vi "Upload Firmware.vi"(5 "Progress Bar":refnum<vi>, 7 "COM Port":refnum<visa-resource-name>="COM5", 8 "Error In":errorcluster, 9 "Firmware Index":u16(ring) items=["LINX -  Serial / USB", "LINX -  Serial / USB [Debug] "], 10 "Device Index":u16=1, 11 "Family Index":T1=1 items=["Arduino", "Digilent", "PJRC"]) -> (0 "Error Out":errorcluster={"status"=TRUE, "code"=-1073807346, "source"="VISA Open in LVH-LINX.lvlib:Upload Firmware.vi"}, 1 "Log Path":path)   [LabVIEW 2014, in "LMH-LINX.lvlib"]
uses:
  <vilib>/MakerHub/LINX/LMH-LINX.lvlib
  <vilib>/MakerHub/LINX/Private/Type Defs/Device Family.ctl
  <vilib>/MakerHub/LINX/Private/Type Defs/All Firmware Data FGV States.ctl
  <vilib>/regexp/Match Regular Expression.xnode
  <vilib>/MakerHub/Toolbox/LMH-Toolbox.lvlib
  <vilib>/MakerHub/LINX/Private/Device/Device.lvlib
panel:
  out "Success?":bool
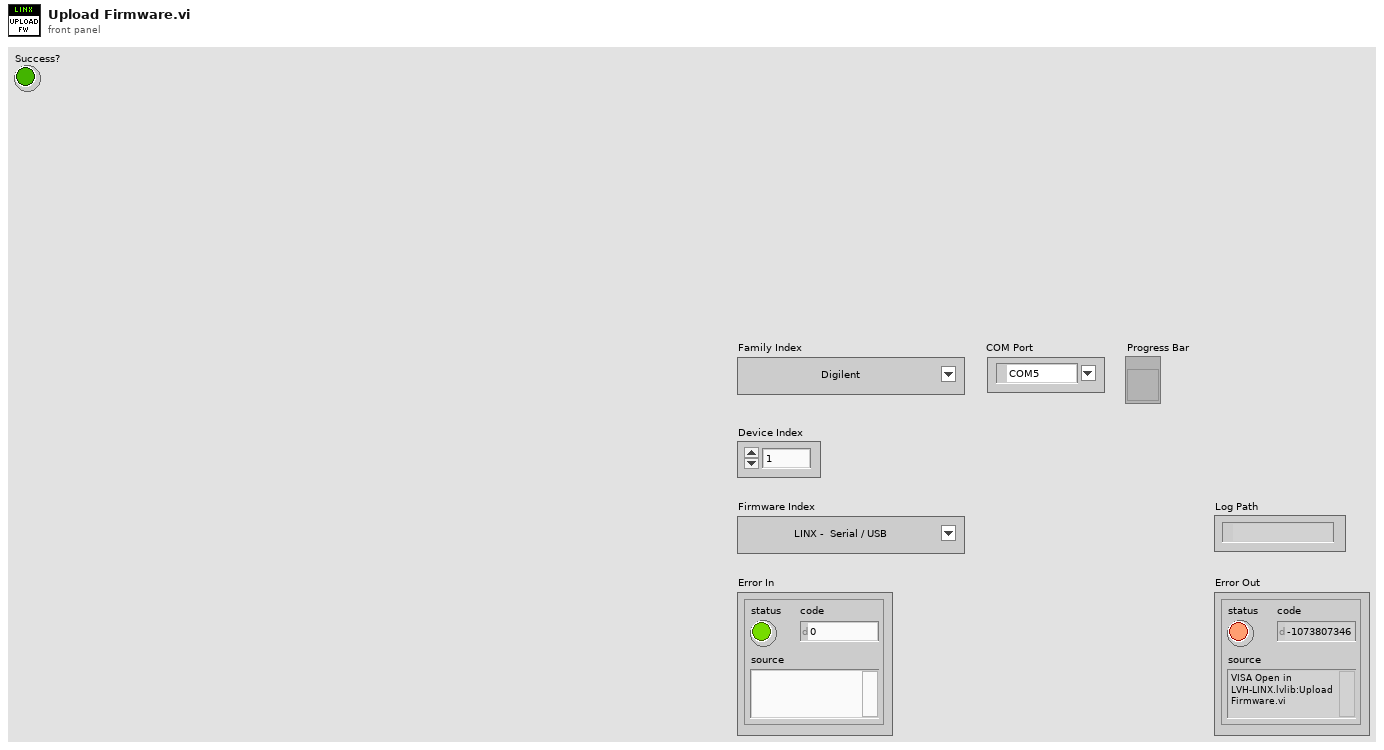
[diagram p1: front panel]
types:
  T1 = typedef "LMH-LINX.lvlib/Device Family.ctl" = u8
  T2 = typedef "LMH-LINX.lvlib/All Firmware Data FGV States.ctl" = enum16{"Set", "Get"}
  T3 = typedef "LMH-LINX.lvlib/Device Firmware.ctl" = cluster{"Firmware Name":string, "Firmware Path":path, "Description":string, "LINX Interface":string, "Flash Util Working Dir":path, "Flash Util Name":string, "Flash Util Args":string, "Flash Timeout (ms)":i32, "Pre-Built Firmware":string, "Build with Arduino IDE":string}
  T4 = typedef "LMH-LINX.lvlib/Device Data.ctl" = cluster{"Family ID":i32, "Family Name":string, "Device ID":i32, "Device Name":string, "Firmware Program Interfaces":string[], "Path":path}
  T5 = typedef "LVDateTimeRec.ctl" = cluster{"fractional second":dbl, "second":i32, "minute":i32, "hour":i32, "day of month":i32, "month":i32, "year":i32, "day of week":i32, "day of year":i32, "DST":i32}
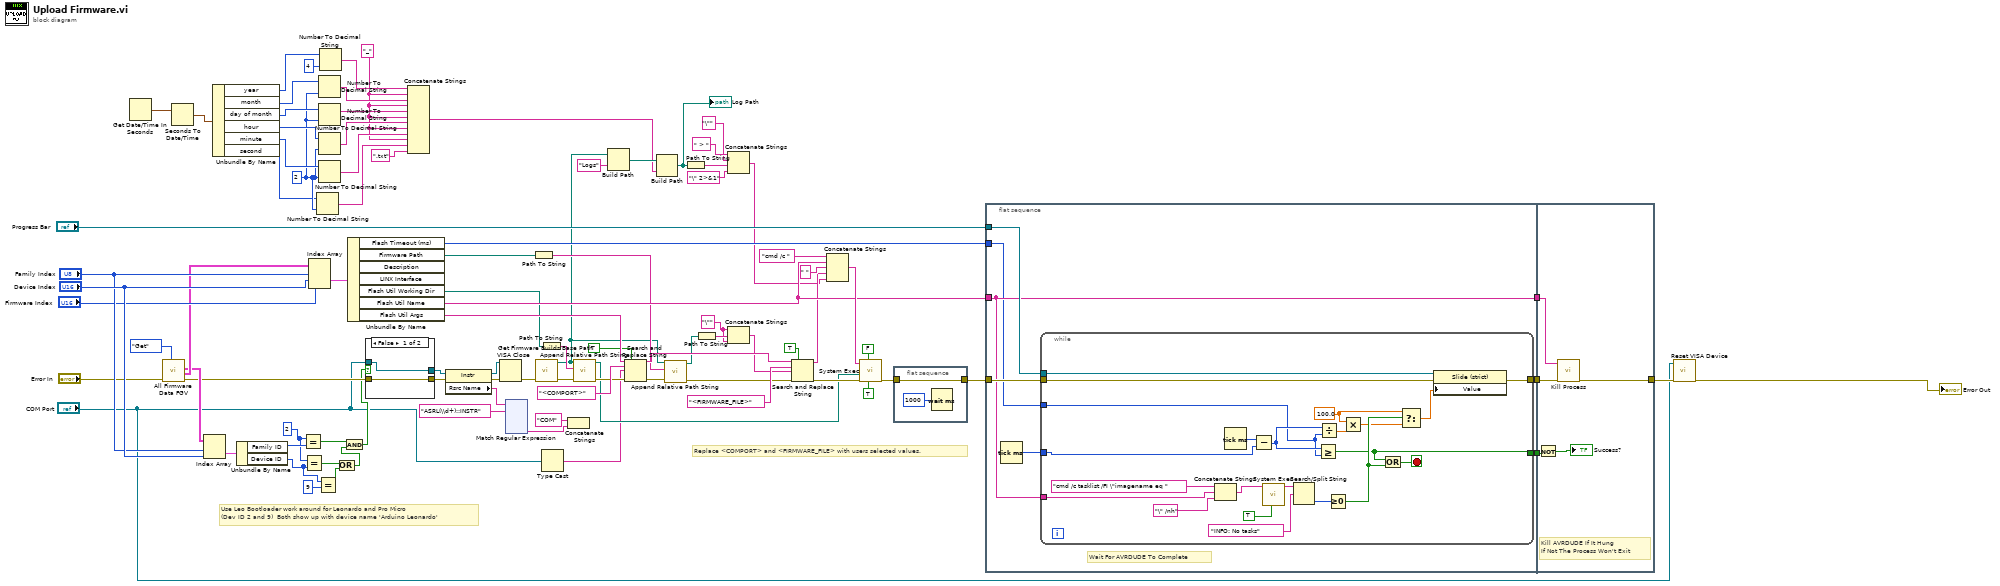
[diagram p0: block diagram]
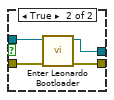
[diagram p2: hidden frame]
diagram:
  w17 = "_" ("string")
  w21 = i16 2 ("width (-)")
  w48 = 2 ("x")
  w54 = "\"" ("string")
  # "Use Leo Bootloader work around for Leonardo and Pro Micro\n(Dev ID 2 and 9)  Both show up with device name 'Arduino Leonardo'"
  # "Replace <COMPORT> and <FIRMWARE_FILE> with users selected values."
  n1 = Get Date/Time In Seconds() -> (seconds since 1Jan1904=w37:timestamp)
  n2 = call <vilib>:"All Firmware Data FGV.vi"("All Firmware Data FGV States"=All_Firmware_Data_FGV_States."Get", "Error In"="Error In") -> ("Error Out"=w46:errorcluster, "Firmwares"=w84:T3[][][], "Devices"=w51:T4[][])  [unwired: 6 in, 1 out]
  n3 = Seconds To Date/Time(time stamp (now)=w37) -> (date time rec=w38:T5)  [unwired: 1 in]
  n4 = Index Array(array=w51, index (row)="Family Index", index (col)="Device Index") -> (element=w50:T4)
  n5 = Unbundle By Name(w38) -> ("year"=w36:i32, "month"=w35:i32, "day of month"=w34:i32, "hour"=w33:i32, "minute"=w32:i32, "second"=w20:i32)
  n6 = Unbundle By Name(w50) -> ("Family ID"=w49:i32, "Device ID"=w14:i32)
  n7 = Equal?(x=w48, y=w49) -> (x = y?=w47:bool)
  n8 = Equal?(x=w48, y=w14) -> (x = y?=w16:bool)
  n9 = Index Array(array=w84, index (dim 0)="Family Index", index (dim 1)="Device Index", index (dim 2)="Firmware Index") -> (element=w83:T3)
  n10 = Number To Decimal String(number=w20, width (-)=w21) -> (decimal integer string=w18:string)
  n11 = Equal?(x=w14, y=9 ("x")) -> (x = y?=w13:bool)
  n12 = Number To Decimal String(number=w35, width (-)=w21) -> (decimal integer string=w29:string)
  n13 = Number To Decimal String(number=w34, width (-)=w21) -> (decimal integer string=w28:string)
  n14 = Number To Decimal String(number=w33, width (-)=w21) -> (decimal integer string=w27:string)
  n15 = Number To Decimal String(number=w32, width (-)=w21) -> (decimal integer string=w26:string)
  n16 = Number To Decimal String(number=w36, width (-)=i16 4) -> (decimal integer string=w30:string)
  n17 = Or(x=w16, y=w13) -> (x .or. y?=w12:bool)
  n18 = And(x=w47, y=w12) -> (x .and. y?=w45:bool)
  n19 = Unbundle By Name(w83) -> ("Flash Timeout (ms)"=w52:i32, "Firmware Path"=w67:path, "Flash Util Working Dir"=w59:path, "Flash Util Name"=w71:string, "Flash Util Args"=w77:string)  [unwired: 2 out]
  n20 = case shown="False" w45 {
    tunnel: [w95 w100] -> w10
    tunnel: w46 -> [w95 w99]
    tunnel: [w96 w98] -> w11
    tunnel: "COM Port" -> [w96 w97]
    frame False {
    }
    frame True {
      n21 = call <vilib>:"Enter Leonardo Bootloader.vi"("Error In"=w99, "VISA resource name"=w97) -> ("Error Out"=w100:errorcluster, "VISA resource name"=w98:refnum<visa-resource-name>)  [unwired: 7 in, 1 out]
    }
  }
  n22 = Concatenate Strings(w30, w17, w29, w17, w28, w17, w27, w17, w26, w17, w18, ".txt" ("string")) -> (w25:string)
  n23 = property class="Instr"(reference=w11, error in=w10) -> (reference out=w8:refnum<visa-resource-name>, error out=w9:errorcluster, "Rsrc Name"=w5:string)
  n24 = VISA Close(VISA resource name=w8, error in (no error)=w9) -> (error out=w7:errorcluster)
  n25 = xnode "Match Regular Expression"("input string"=w5, "regular expression"="ASRL(\\d+)::INSTR") -> ("submatch 1"=w3:string)  [unwired: 4 in, 5 out]
  n26 = Path To String(path=w67) -> (string=w65:string)
  n27 = call <vilib>:"Get Firmware Builds Base Path.vi"("Error In"=w7) -> ("Error Out"=w61:errorcluster, "Firmware Builds Base Path"=w44:path)  [unwired: 9 in]
  n28 = Path To String(path=w59) -> (string=w58:string)
  n29 = Type Cast(x="COM Port") -> (*(type *) &x=w1:string)  [unwired: 1 in]
  n30 = Concatenate Strings("COM" ("string"), w3) -> ()  [unwired: 1 out]
  n31 = call <vilib>:"Append Relative Path String.vi"("Error In"=w61, "Relative Path"=w58, "Base Path"=w44) -> ("Error Out"=w60:errorcluster, "Absolute Path"=w57:path)  [unwired: 7 in]
  n32 = Build Path(base path=w44, name or relative path="Logs") -> (appended path=w42:path)
  n33 = Search and Replace String(replace all?=TRUE ("replace all? (F)"), input string=w77, search string="<COMPORT>", replace string=w1, error in=w60) -> (result string=w68:string, error out=w53:errorcluster)  [unwired: 3 in, 2 out]
  n34 = Build Path(base path=w42, name or relative path=w25) -> (appended path=w41:path)
  "Log Path" <- w41
  n35 = call <vilib>:"Append Relative Path String.vi"("Error In"=w53, "Relative Path"=w65, "Base Path"=w44) -> ("Error Out"=w63:errorcluster, "Absolute Path"=w64:path)  [unwired: 7 in]
  n36 = Path To String(path=w41) -> (string=w24:string)
  n37 = Path To String(path=w64) -> (string=w55:string)
  n38 = Concatenate Strings(" > " ("string"), "\"" ("string"), w24, "\" 2>&1" ("string")) -> (w39:string)
  n39 = Concatenate Strings(w54, w55, w54) -> (w56:string)
  n40 = Search and Replace String(replace all?=TRUE ("replace all? (F)"), input string=w68, search string="<FIRMWARE_FILE>", replace string=w56, error in=w63) -> (result string=w66:string, error out=w62:errorcluster)  [unwired: 3 in, 2 out]
  n41 = Concatenate Strings("cmd /c " ("string"), w71, " " ("string"), w66, w39) -> (w74:string)
  n42 = call <vilib>:"System Exec.vi"("run minimized? (F)"=TRUE, "wait until completion? (T)"=FALSE, "error in (no error)"=w62, "working directory"=w57, "command line"=w74) -> ("error out"=w80:errorcluster)  [unwired: 3 in, 3 out]
  n43 = flat-sequence {
    tunnel: [w102] -> w72
    tunnel: w80 -> [w102]
    frame #0 {
      n44 = Wait (ms)(milliseconds to wait=u32 1000) -> ()  [unwired: 1 out]
    }
  }
  n45 = flat-sequence {
    tunnel: w72 -> [w107]
    tunnel: [w108] -> w88
    tunnel: "Progress Bar" -> [w106]
    tunnel: [w105] -> w87
    tunnel: w71 -> [w104]
    tunnel: [w104] -> w86
    tunnel: w52 -> [w103]
    tunnel: w88 -> [w136]
    tunnel: [w135] -> w73
    tunnel: w87 -> [w134]
    tunnel: w86 -> [w132]
    frame #0 {
      # "Wait For AVRDUDE To Complete"
      n46 = Tick Count (ms)() -> (millisecond timer value=w109:u32)
      n47 = while {
        tunnel: w109 -> [w130]
        tunnel: [w129] -> w108
        tunnel: w107 -> [w128]
        tunnel: w106 -> [w127]
        tunnel: [w115] -> w105
        tunnel: w104 -> [w111]
        tunnel: w103 -> [w110]
        stop <- w121 stop-if-true
        w118 = 100.0 ("x")
        n48 = Concatenate Strings("cmd /c tasklist /FI \"imagename eq " ("command line"), w111, "\" /nh" ("string")) -> (w113:string)
        n49 = Tick Count (ms)() -> (millisecond timer value=w131:u32)
        n50 = Subtract(x=w131, y=w130) -> (x-y=w126:u32)
        n51 = call <vilib>:"System Exec.vi"("run minimized? (F)"=TRUE, "command line"=w113) -> ("standard output"=w123:string)  [unwired: 6 in, 3 out]
        n52 = Search/Split String(string=w123, search string/char (-)="INFO: No tasks") -> (offset of match=w120:i32)  [unwired: 1 in, 2 out]
        n53 = Greater Or Equal?(x=w126, y=w110) -> (x >= y?=w115:bool)
        n54 = Divide(x=w126, y=w110) -> (x/y=w125:dbl)
        n55 = Greater Or Equal To 0?(x=w120) -> (x >= 0?=w119:bool)
        n56 = Multiply(x=w118, y=w125) -> (x*y=w117:dbl)
        n57 = Or(x=w115, y=w119) -> (x .or. y?=w121:bool)
        n58 = Select(t=w118, s=w119, f=w117) -> (s? t:f=w116:dbl)
        n59 = property class="Slide (strict)"(reference=w127, error in=w128, "Value"=w116) -> (error out=w129:errorcluster)  [unwired: 1 out]
      }
    }
    frame #1 {
      # "Kill AVRDUDE If It Hung\nIf Not The Process Won't Exit"
      n60 = Not(x=w134) -> (.not. x?=→"Success?":bool)
      n61 = call <vilib>:"Kill Process.vi"("Error In"=w136, "Process Name"=w132) -> ("Error Out"=w135:errorcluster)  [unwired: 9 in]
    }
  }
  n62 = call <vilib>:"Reset VISA Device.vi"("Error In"=w73, "VISA resource name"="COM Port") -> ("Error Out"=→"Error Out":errorcluster)  [unwired: 9 in]
